vi "ArrDevMeasAction.vi"(6 "Scan":bool, 7 "DevId":i32, 8 "error in (no error)":errorcluster caption="entrée d'erreur (pas d'erreur)", 9 "CurvePointIndex":i32, 10 "AllPointIndex":i32, 11 "Device In":refnum<class "RedTide650.lvclass"> caption="DNL_LabVIEW Object in") -> (0 "error out":errorcluster caption="sortie d'erreur", 1 "ArrDevDat":T1[](array[typedef]), 2 "ArrDevDatOut":dbl[][](array[numeric]), 3 "Device Out":refnum<class "RedTide650.lvclass"> caption="DNL_LabVIEW Object out", 5 "MeasOut":dbl[](array[numeric]))   [LabVIEW 2019, in "RedTide650.lvclass"]
uses:
  RedTide650.lvclass
  C:/Programmes Labview/LabscanV1A/DevicesClass/BaseDevice/BaseDevice.lvclass
  Experiment Class/ArrDevData.ctl
  RedTide650.lvclass/RedTide650.ctl
  <vilib>/Utility/error.llb/Error Cluster From Error Code.vi
  <vilib>/ErrorRing/Error Ring.xnode
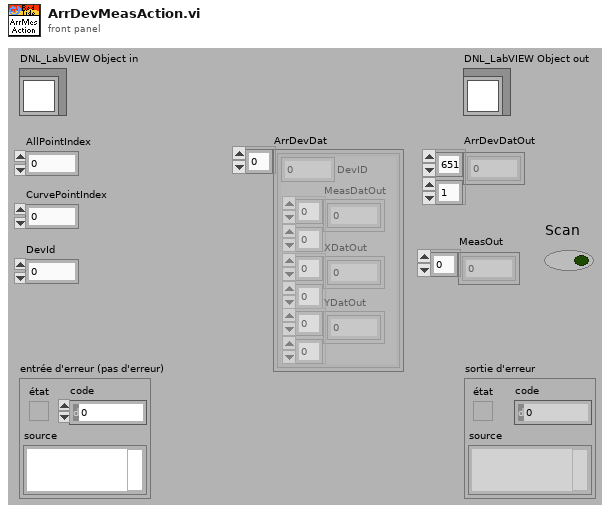
[diagram p1: front panel]
types:
  T1 = typedef "ArrDevData.ctl" = cluster{"MeasDatOut":dbl[][], "XDatOut":dbl[][], "YDatOut":dbl[][], "DevID":i32}
  T2 = typedef "RedTide650.lvclass/RedTide650_Func.ctl" = enum16{"ReadSpectrum (Acq)"}
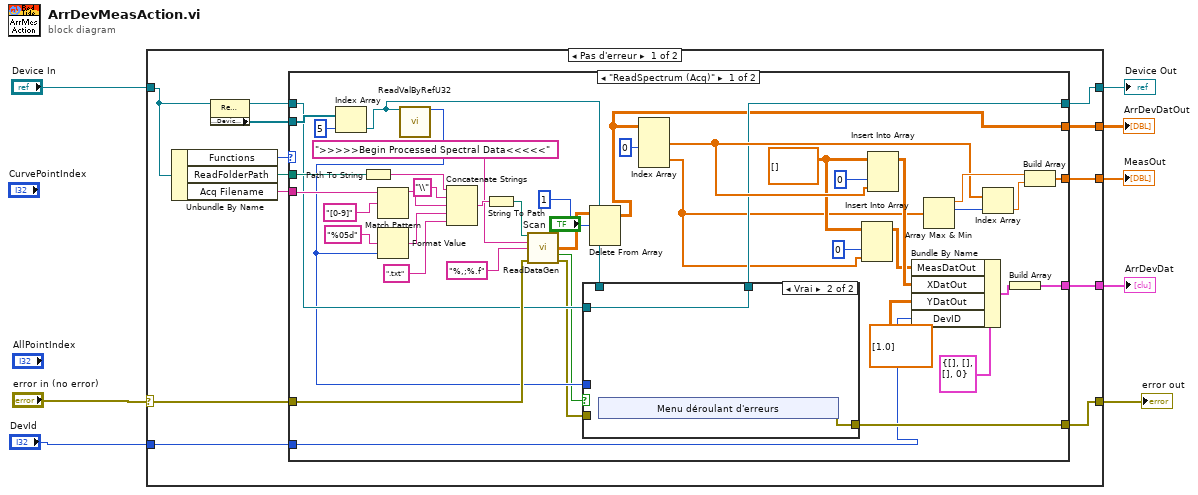
[diagram p0: block diagram]
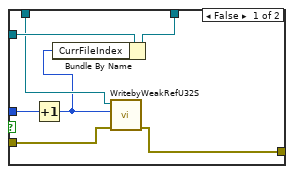
[diagram p2: hidden frame]
diagram:
  n1 = case shown="Pas d'erreur" "error in (no error)" {
    selector: "error in (no error)" -> [w20 w81]
    tunnel: [w13 w82] -> w7
    tunnel: "Device In" -> [w12 w82]
    tunnel: [w21 w81] -> w5
    tunnel: [w18 _] -> w4
    tunnel: [w17 _] -> w3
    tunnel: [w16 _] -> w2
    tunnel: "DevId" -> [w9 _]
    frame No Error {
      n2 = Unbundle By Name(w12) -> ("Functions"=w19:T2, "ReadFolderPath"=w15:path, "Acq Filename"=w14:string)
      n3 = property class="RedTide650.lvclass"(reference=w12) -> (reference out=w11:refnum<class "RedTide650.lvclass">, "Accessor:DeviceCtrl"=w10:refnum<vi>[])  [unwired: 1 in, 1 out]
      n4 = case shown="\"ReadSpectrum (Acq)\"" w19 {
        tunnel: [w36 w80] -> w21
        tunnel: w20 -> [w51 w80]
        tunnel: [w44 _] -> w18
        tunnel: [w22 _] -> w17
        tunnel: [w62 _] -> w16
        tunnel: w15 -> [w57 _]
        tunnel: w14 -> [w60 _]
        tunnel: [w34 w79] -> w13
        tunnel: w11 -> [w35 w79]
        tunnel: w10 -> [w38 _]
        tunnel: w9 -> [w24 _]
        frame "ReadSpectrum (Acq)" {
          w27 = dbl[][] [] ("tableau")
          n5 = Index Array(array=w38, index=5 ("indice")) -> (element=w31:refnum<vi>)
          n6 = Path To String(path=w57) -> (string=w56:string)
          n7 = Match Pattern(string=w60, regular expression="[0-9]" ("expression régulière")) -> (before substring=w40:string)  [unwired: 1 in, 3 out]
          n8 = call <userlib>:"ReadValByRefU32.vi"("Control Ref"=w31) -> ("Valeur"=w32:u32)  [unwired: 13 in, 1 out]
          n9 = Format Value(format string="%05d" ("chaîne de format"), value (0)=w32) -> (output string=w59:string)  [unwired: 1 in]
          n10 = Concatenate Strings(w56, "\\" ("chaîne"), w40, w59, ".txt" ("chaîne")) -> (w55:string)
          n11 = String To Path(string=w55) -> (path=w54:path)
          n12 = call <userlib>:"ReadDataGen.vi"("path"=w54, "header end"=">>>>>Begin Processed Spectral Data<<<<<", "chaîne de format"="%,;%.f", "error in (no error)"=w51) -> ("Scan Data"=w46:dbl[][], "ReadError"=w29:bool, "error out"=w30:errorcluster)  [unwired: 7 in, 2 out]
          n13 = case shown="Vrai" w29 {
            tunnel: [w66 w72] -> w36
            tunnel: w31 -> [w68 _]
            tunnel: w32 -> [w71 _]
            tunnel: w35 -> [w70 w73]
            tunnel: [w69 w73] -> w34
            tunnel: w30 -> [w65 _]
            frame False {
              n14 = Increment(x=w71) -> (x+1=w67:u32)
              n15 = Bundle By Name(cluster=w70, "CurrFileIndex"=w67) -> (w69:refnum<class "RedTide650.lvclass">)
              n16 = call <userlib>:"WritebyWeakRefU32S.vi"("error in"=w65, "Valeur"=w67, "Control Ref"=w68) -> ("error out"=w66:errorcluster)  [unwired: 8 in]
            }
            frame True {
              n17 = xnode "Menu déroulant d'erreurs"() -> ("sortie d'erreur"=w72:errorcluster)
            }
          }
          n18 = Delete From Array(array=w46, length=1 ("longueur")) -> (array with subset deleted=w22:dbl[][])  [unwired: 2 in, 1 out]
          n19 = Index Array(array=w22, index (col) #1=0 ("indice désactivé (col)")) -> (element #1=w42:dbl[], element #2=w26:dbl[])  [unwired: 3 in]
          n20 = Insert Into Array(array=w27, index (col)=0 ("indice désactivé (col)"), new element=w26) -> (w25:dbl[][])  [unwired: 1 in]
          n21 = Insert Into Array(array=w27, index (col)=0 ("indice désactivé (col)"), new element=w42) -> (w48:dbl[][])  [unwired: 1 in]
          n22 = Bundle By Name(cluster=T1 {"MeasDatOut"=[], "XDatOut"=[], "YDatOut"=[], "DevID"=0} ("cluster de sortie"), "MeasDatOut"=w25, "XDatOut"=w48, "YDatOut"=dbl[][] [[1.0]], "DevID"=w24) -> (w63:T1)
          n23 = Array Max & Min(array=w26) -> (max value=w45:dbl, max index (indices)=w41:i32)  [unwired: 2 out]
          n24 = Index Array(array=w42, index=w41) -> (element=w43:dbl)
          n25 = Build Array(w63) -> (w62:T1[])
          n26 = Build Array(w45, w43) -> (w44:dbl[])
        }
        frame Default {
        }
      }
    }
    frame Error {
    }
  }
  "error out" <- w5
  "Device Out" <- w7
  "ArrDevDatOut" <- w3
  "ArrDevDat" <- w2
  "MeasOut" <- w4
